vi "Target.vi"() -> ()   [LabVIEW 2025]
uses:
  <vilib>/Platform/TimedLoop/XDataNode/timing_clust.ctl
  <vilib>/Platform/TimedLoop/XDataNode/nitl_modes.ctl
  <vilib>/Platform/TimedLoop/XDataNode/wakeup.ctl
  <vilib>/rvi/Emulation/niFpgaSctlEmulationGetInTimedLoop.vi
  <vilib>/rvi/Emulation/niFpgaEmulationReportErrorSimple.vi
  <vilib>/rvi/Emulation/niFpgaGetClockAttributes.vi
  <vilib>/rvi/Emulation/niFpgaCriticalErrorInLSC.vi
  <vilib>/rvi/linearAlgebra/MatrixMultiply/simVIs/SubVI/nifxpla_MatrixMultiply_SimMatrixSizes.vi
  <vilib>/rvi/linearAlgebra/MatrixMultiply/simVIs/SubVI/nifxpla_MatrixMultiply_Sim4WireAdapterVector.vi
  <vilib>/rvi/linearAlgebra/MatrixMultiply/simVIs/SubVI/nifxpla_MatrixMultiply_SimFrameHandShake.vi
  <vilib>/rvi/linearAlgebra/MatrixMultiply/simVIs/SubVI/nifxpla_MatrixMultiply_SimEndlessCounter.vi
  <vilib>/rvi/linearAlgebra/MatrixMultiply/simVIs/SubVI/nifxpla_MatrixMultiply_SimVectorDataBuffer.vi
  <vilib>/rvi/ClientSDK/Core/DevComputerLib/Private/Multiply(dfxp64).vi
  <vilib>/rvi/ClientSDK/Core/DevComputerLib/Private/Dfxp128ToDfxp256.vi
  <vilib>/rvi/ClientSDK/Core/DevComputerLib/Private/Add(dfxp256).vi
  <vilib>/rvi/ClientSDK/Core/DevComputerLib/Private/Subtract(dfxp256).vi
  <vilib>/rvi/ClientSDK/Core/DevComputerLib/Private/ToDfxp64(dfxp256).vi
  <vilib>/platform/TimedLoop/XDataNode/XDataNode.xnode
  <vilib>/rvi/linearAlgebra/MatrixMultiply/XNode/nifxpla_MatrixMultiply.xnode
  <vilib>/rvi/linearAlgebra/MatrixMultiply/simVIs/nifxpla_MatrixMultiply_SimTemplateEinEout.vi
  <vilib>/rvi/linearAlgebra/MatrixMultiply/simVIs/nifxpla_MatrixMultiply_SimTemplateEinVout.vi
  <vilib>/rvi/linearAlgebra/MatrixMultiply/simVIs/nifxpla_MatrixMultiply_SimTemplateVinEout.vi
  <vilib>/rvi/linearAlgebra/MatrixMultiply/simVIs/nifxpla_MatrixMultiply_SimTemplateVinVout.vi
  <vilib>/Platform/TimedLoop/XDataNode/XDNodeRunTimeDep.lvlib
panel:
  out "C":fxp<+/-,32,16>[](array[numeric])
  out "Cycle Count":i32
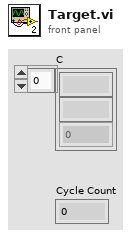
[diagram p1: front panel]
types:
  T1 = typedef "XDNodeRunTimeDep.lvlib/timing_clust.ctl" = cluster{"Expected End [f-1]":u64, "Actual End [f-1]":u64, "Finished Late? [f-1]":bool, "Expected End [i-1]":u64, "Actual End [i-1]":u64, "Finished Late? [i-1]":bool, "Expected Start [i]":u64, "Actual Start [i]":u64, "Expected Start [f]":u64, "Actual Start [f]":u64, "Source Name":string, "Structure Name":string, "Period":i64, "Deadline":i64, "Offset":i64, "Start":i64, "Priority":i32, "Timeout":i32, "Mode":T2, "Wakeup Reason":T3, "Error":errorcluster, "Source Type":string, "Secondary Source Type":string, "Global End Time":u64, "Global Start Time":u64, "Frame Duration":u64, "Iteration Duration":u64, "Assigned CPU":i32, "I/O Scan Engine Mode":u32}
  T2 = typedef "XDNodeRunTimeDep.lvlib/nitl_modes.ctl" = enum32{"No Change", "Process missed periods, maintain original phase", "Discard missed periods, maintain original phase", "Process missed periods, ignore original phase", "Discard missed periods, ignore original phase"}
  T3 = typedef "XDNodeRunTimeDep.lvlib/wakeup.ctl" = enum32{"Normal", "Aborted", "Asynchronous wakeup", "Timing source error", "Timed loop error", "Timeout"}
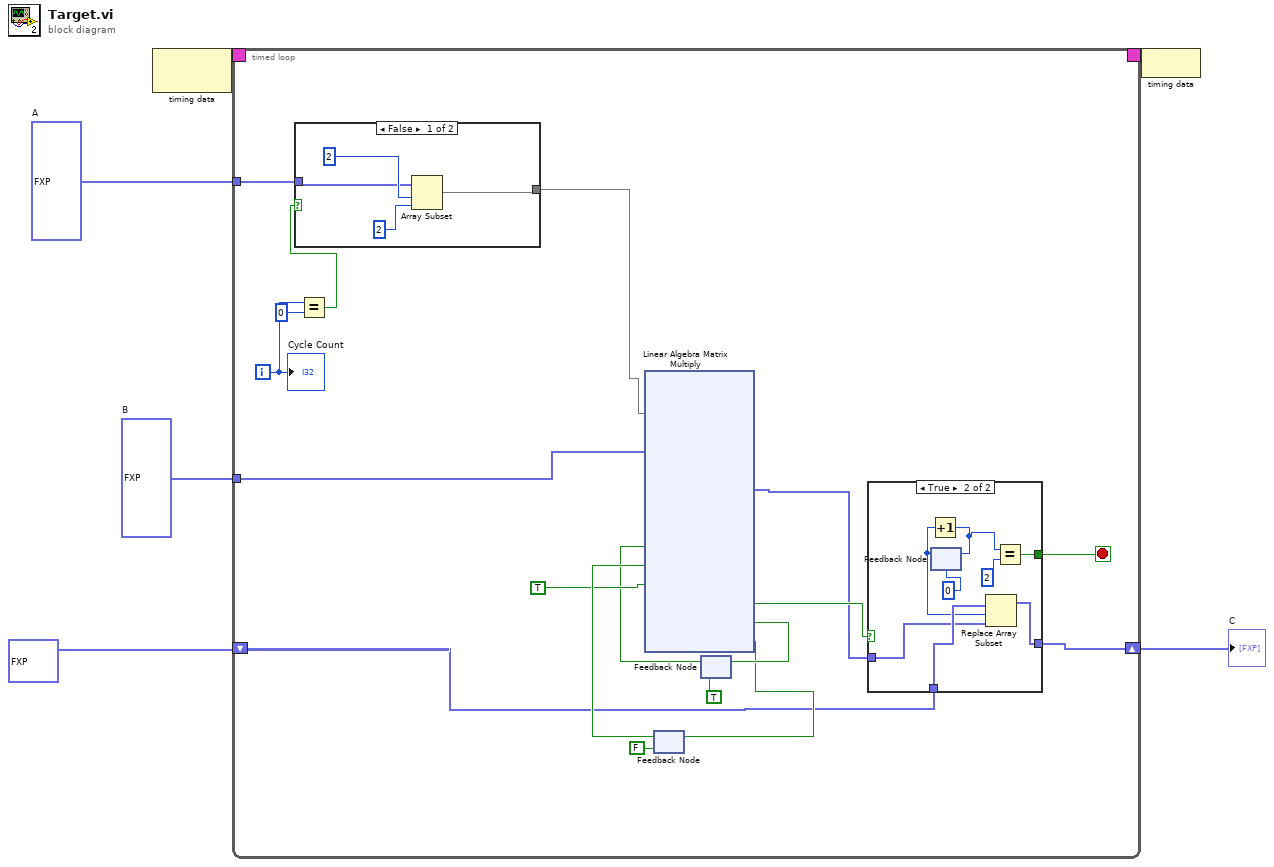
[diagram p0: block diagram]
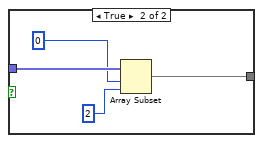
[diagram p2: hidden frame]
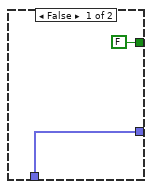
[diagram p3: hidden frame]
diagram:
  w2 = fxp<+/-,32,16>[] [1.0, 2.0, 3.0, 4.0]  # A
  w3 = fxp<+/-,32,16>[] [1.0, 2.0]  # B
  n1 = node-c288() -> (w6:T1)  [unwired: 1 in]
  n2 = timed-loop {
    timing: w6 -> [_]
    timing-out: [_] -> w5
    shift-right: [w16] -> w1
    shift-left: fxp<+/-,32,16>[] [0.0, 0.0] -> [w15]
    tunnel: w3 -> [w13]
    tunnel: w2 -> [w11]
    i -> [w9]
    stop <- w14 stop-if-true
    n3 = Equal?(x=w9, y=0) -> (x = y?=w7:bool)
    n4 = case shown="False" w7 {
      tunnel: w11 -> [w26 w32]
      tunnel: [w25 w30] -> w10
      frame False {
        n5 = Array Subset(array=w26, index=2 ("length"), length=2) -> (w25:fxp<+/-,32,16>[])
      }
      frame True {
        n6 = Array Subset(array=w32, index=0 ("length"), length=2) -> (w30:fxp<+/-,32,16>[])
      }
    }
    n7 = feedback #1(FALSE ("ready for b")) -> (w22:bool)
    n8 = feedback #2(TRUE ("ready for a")) -> (w12:bool)
    n9 = xnode ("Linear Algebra Matrix Multiply")("ar"=w10, "br"=w13, "a valid"=w12, "b valid"=w22, "ready for output (T)"=TRUE) -> ("cr"=w17:fxp<+/-,32,16>[], "output valid"=w18:bool, "ready for a"=w24:bool, "ready for b"=w23:bool)  [unwired: 2 in, 2 out]
    n10 = feedback-in #1(w23) -> ()
    n11 = feedback-in #2(w24) -> ()
    n12 = case shown="True" w18 {
      tunnel: w17 -> [_ w37]
      tunnel: [w34 w41] -> w16
      tunnel: w15 -> [w34 w42]
      tunnel: [FALSE w38] -> w14
      frame False {
      }
      frame True {
        n13 = feedback #3(0 ("x")) -> (w36:i32)
        n14 = Increment(x=w36) -> (x+1=w35:i32)
        n15 = feedback-in #3(w35) -> ()
        n16 = Replace Array Subset(array=w42, new element=w37, index=w36) -> (w41:fxp<+/-,32,16>[])
        n17 = Equal?(x=w35, y=2) -> (x = y?=w38:bool)
      }
    }
    "Cycle Count" <- w9
  }
  "C" <- w1
  n18 = node-c288(w5) -> ()
